vi "ToscaCal-Compute ASTF.vi"(0 "Mag":dbl[][](array[numeric]), 1 "Stimulus":dbl[](array[numeric]), 5 "Phase":dbl[][](array[numeric]), 7 "df (Hz)":dbl, 9 "Mic Gain (dB)":dbl=50000.0, 11 "error in (no error)":errorcluster, 12 "Attenuation (dB)":dbl, 13 "Compute Options":T1={"Smooth?"=FALSE, "Cal Mic Sens"=-146.12351367888365, "UseMicCal"=FALSE, "Path"=path ""} {"Cal Mic Sens" format="%.2f"}) -> (4 "ASTF Mag":dbl[](array[numeric]), 6 "ASTF Phase":dbl[](array[numeric]), 8 "Frequency":dbl[](array[numeric]), 15 "error out":errorcluster)   [LabVIEW 2020]
uses:
  ToscaCal-Computation Options.ctl
  epl-vi-lib/Utility VIs/Math VIs/LinSpace (x0-dx-npts).vi
  epl-vi-lib/Utility VIs/Math VIs/FFT x(t) to dB,Degrees (1D).vi
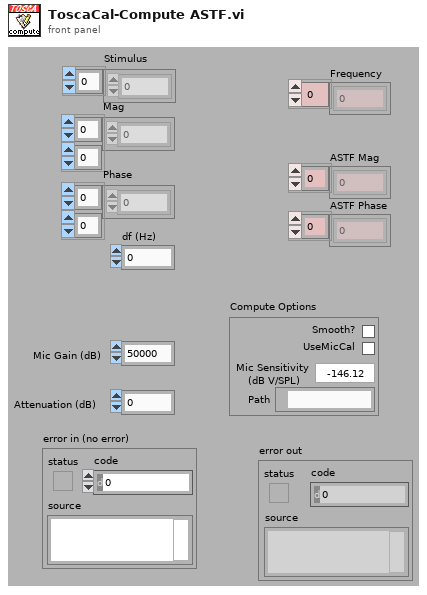
[diagram p1: front panel]
types:
  T1 = typedef "ToscaCal-Computation Options.ctl" = cluster{"Smooth?":bool, "Cal Mic Sens":dbl, "UseMicCal":bool, "Path":path}
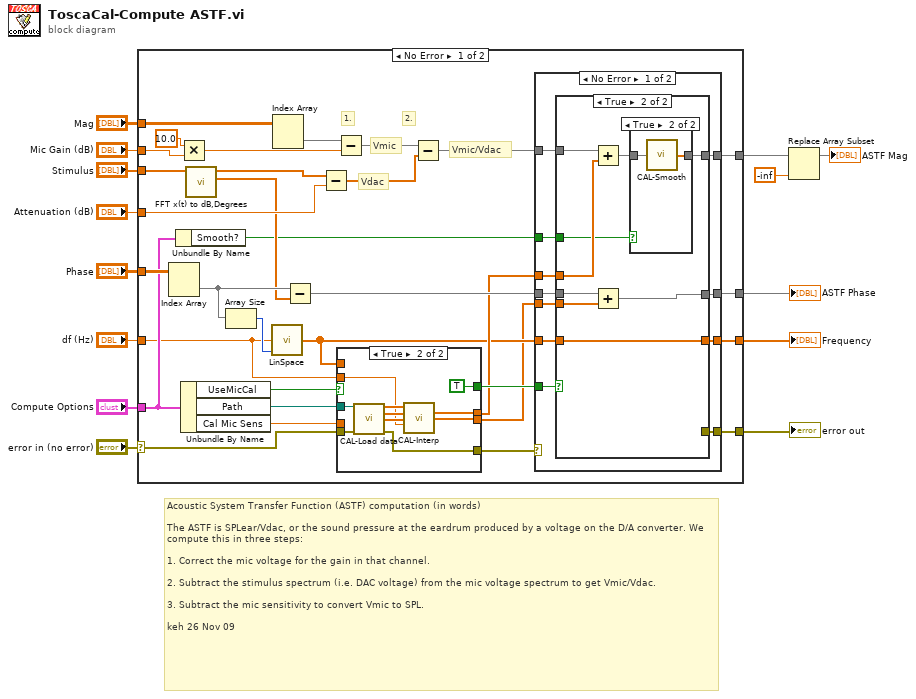
[diagram p0: block diagram]
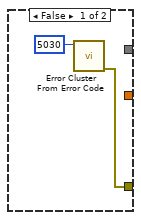
[diagram p2: hidden frame]
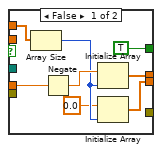
[diagram p5: hidden frame]
diagram:
  # "Acoustic System Transfer Function (ASTF) computation (in words)\n\nThe ASTF is SPLear/Vdac, or the sound pressure at the eardrum produced by a voltage on the D/A converter. We compute this in three steps:\n\n1. Correct the mic voltage for the gain in that channel.\n\n2. Subtract the stimulus spectrum (i.e. DAC voltage) from the mic voltage spectrum to get Vmic/Vdac.\n\n3. Subtract the mic sensitivity to convert Vmic to SPL.\n\nkeh 26 Nov 09"
  n1 = case shown="No Error" "error in (no error)" {
    selector: "error in (no error)" -> [w30 w91]
    tunnel: "Mag" -> [w46 _]
    tunnel: "Phase" -> [w45 _]
    tunnel: [w34 _] -> w12
    tunnel: [w24 _] -> w11
    tunnel: "Stimulus" -> [w41 _]
    tunnel: "df (Hz)" -> [w15 _]
    tunnel: [w19 _] -> w7
    tunnel: "Mic Gain (dB)" -> [w37 _]
    tunnel: [w21 w91] -> w5
    tunnel: "Attenuation (dB)" -> [w42 _]
    tunnel: "Compute Options" -> [w17 _]
    frame No Error {
      # "2."
      # "1."
      # "Vmic/Vdac"
      # "Vdac"
      # "Vmic"
      n2 = Index Array(array=w45) -> (element=w44:dbl[])  [unwired: 2 in]
      n3 = Unbundle By Name(w17) -> ("Smooth?"=w16:bool)
      n4 = Multiply(x=10.0, y=w37) -> (x*y=w38:dbl)
      n5 = Unbundle By Name(w17) -> ("UseMicCal"=w29:bool, "Path"=w28:path, "Cal Mic Sens"=w27:dbl)
      n6 = call-poly "FFT x(t) to dB,Degrees.vi"("X"=w41) -> ("+Freq Phase of FFT (degrees)"=w40:dbl[], "+Freq. Mag of FFT (dB rms)"=w39:dbl[])  [unwired: 8 in, 1 out]
      n7 = Array Size(array=w44) -> (size(s)=w43:i32)
      n8 = call-poly "LinSpace.vi"("npts"=w43, "dx"=w15) -> ("Array"=w20:dbl[])  [unwired: 2 in, 1 out]
      n9 = Index Array(array=w46) -> (element=w33:dbl[])  [unwired: 2 in]
      n10 = Subtract(x=w44, y=w40) -> (x-y=w25:dbl[])
      n11 = Subtract(x=w39, y=w42) -> (x-y=w35:dbl[])
      n12 = Subtract(x=w33, y=w38) -> (x-y=w32:dbl[])
      n13 = case shown="True" w29 {
        tunnel: w30 -> [_ w90]
        tunnel: w20 -> [w80 _]
        tunnel: w28 -> [_ w89]
        tunnel: w27 -> [w79 _]
        tunnel: [TRUE ("arrays equal?") TRUE ("arrays equal?")] -> w23
        tunnel: [_ w88] -> w26
        tunnel: [w78 w84] -> w22
        tunnel: [w74 w83] -> w18
        tunnel: w15 -> [_ w82]
        frame False {
          n14 = Array Size(array=w80) -> (size(s)=w76:i32)
          n15 = Negate(x=w79) -> (-x=w77:dbl)
          n16 = Initialize Array(w77, w76) -> (w78:dbl[])
          n17 = Initialize Array(0.0 ("element"), w76) -> (w74:dbl[])
        }
        frame True {
          n18 = call "CAL-Load data.vi"("user path"=w89, "error in (no error)"=w90) -> ("Frequency (Hz)"=w87:dbl[], "Mag"=w86:dbl[], "Phase"=w85:dbl[], "error out"=w88:errorcluster)  [unwired: 6 in, 4 out]
          n19 = call "CAL-Interp.vi"("Frequency (Hz)"=w87, "Magnitude (dB)"=w86, "Phase (degrees)"=w85, "df (Hz)"=w82) -> ("Interp Magnitude (dB)"=w84:dbl[], "Interp Phase (degrees)"=w83:dbl[])  [unwired: 8 in, 2 out]
        }
      }
      n20 = Subtract(x=w32, y=w35) -> (x-y=w31:dbl[])
      n21 = case shown="No Error" w26 {
        selector: w26 -> [_ w72]
        tunnel: w22 -> [w57 _]
        tunnel: [w56 _] -> w34
        tunnel: w31 -> [w55 _]
        tunnel: [w51 w72] -> w21
        tunnel: w25 -> [w53 _]
        tunnel: [w52 _] -> w24
        tunnel: w23 -> [w54 _]
        tunnel: w20 -> [w50 _]
        tunnel: [w49 _] -> w19
        tunnel: w18 -> [w48 _]
        tunnel: w16 -> [w47 _]
        frame No Error {
          n22 = case shown="True" w54 {
            tunnel: w57 -> [_ w68]
            tunnel: [_ w60] -> w56
            tunnel: w55 -> [_ w67]
            tunnel: w53 -> [_ w66]
            tunnel: [_ w65] -> w52
            tunnel: [w59 _] -> w51
            tunnel: w50 -> [_ w64]
            tunnel: [_ w64] -> w49
            tunnel: w48 -> [_ w63]
            tunnel: w47 -> [_ w62]
            frame False {
              n23 = call <vilib>:"Error Cluster From Error Code.vi"("error code (0)"=5030) -> ("error out"=w59:errorcluster)  [unwired: 8 in]
            }
            frame True {
              n24 = Add(x=w67, y=w68) -> (x+y=w61:dbl[])
              n25 = Add(x=w66, y=w63) -> (x+y=w65:dbl[])
              n26 = case shown="True" w62 {
                tunnel: w61 -> [w69 w71]
                tunnel: [w69 w70] -> w60
                frame False {
                }
                frame True {
                  n27 = call "CAL-Smooth.vi"("Magnitude"=w71) -> ("Magnitude Smoothed"=w70:dbl[])
                }
              }
            }
          }
        }
        frame Error {
        }
      }
    }
    frame Error {
    }
  }
  "ASTF Phase" <- w11
  "error out" <- w5
  "Frequency" <- w7
  n28 = Replace Array Subset(array=w12, new element=-inf) -> (→"ASTF Mag":dbl[])  [unwired: 1 in]
